vi "Set VI Refnum.vi"(8 "error in (no error)":errorcluster, 10 "VI Refnum":refnum<vi>, 11 "Sabritas Actor in":refnum<class "Sabritas Actor.lvclass">) -> (0 "error out":errorcluster, 3 "Sabritas Actor out":refnum<class "Sabritas Actor.lvclass">)   [LabVIEW 2020, in "Sabritas Actor.lvlib" / "Sabritas Actor.lvclass"]
uses:
  Sabritas Actor.lvclass
  Sabritas Actor.lvclass/Sabritas Actor.ctl
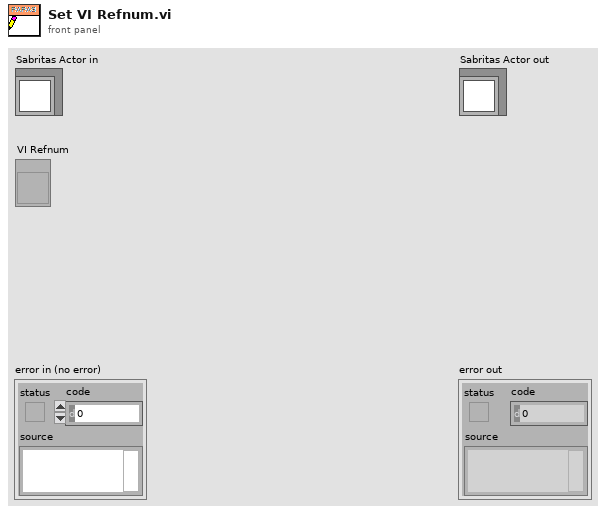
[diagram p1: front panel]
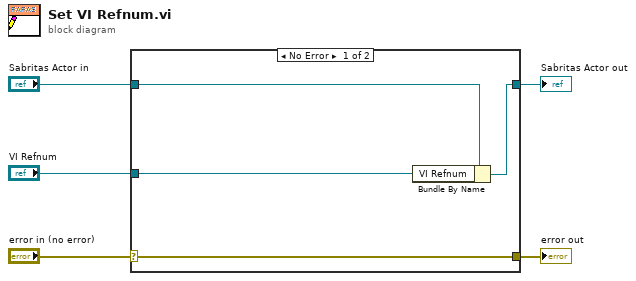
[diagram p0: block diagram]
diagram:
  n1 = case shown="No Error" "error in (no error)" {
    selector: "error in (no error)" -> [w9 w10]
    tunnel: [w9 w10] -> w4
    tunnel: [w7 w11] -> w2
    tunnel: "Sabritas Actor in" -> [w8 w11]
    tunnel: "VI Refnum" -> [w6 _]
    frame No Error {
      n2 = Bundle By Name(cluster=w8, "VI Refnum"=w6) -> (w7:refnum<class "Sabritas Actor.lvclass">)
    }
    frame Error {
    }
  }
  "error out" <- w4
  "Sabritas Actor out" <- w2
